vi "Digital_Bridge_3_kart.vi"() -> ()   [LabVIEW 2014] (continued)
                      frame False {
                        n3107 = local read "X Range KV"() -> (w6899:dbl)
                        n3108 = local read "Y Range KV"() -> (w6898:dbl)
                        n3109 = global write "show_sensitivity.vi" "show sensitivity (kelvin  x)"(w6899) -> ()
                        n3110 = global write "show_sensitivity.vi" "show sensitivity (kelvin  y)"(w6898) -> ()
                      }
                      frame True {
                        w6900 = 10.0 ("Max. Hassasiyet")
                        n3111 = global write "show_sensitivity.vi" "show sensitivity (kelvin  x)"(w6900) -> ()
                        n3112 = global write "show_sensitivity.vi" "show sensitivity (kelvin  y)"(w6900) -> ()
                      }
                    }
                  }
                  frame #6 {
                    n3113 = local write "kelvin switch"(FALSE ("wagner switch")) -> ()
                    n3114 = local write "Start Kelvin X"(TRUE ("START WAGNER")) -> ()
                  }
                }
              }
            }
            n3115 = case shown="True" "RESET SENS X 5" {
              frame False {
              }
              frame True {
                n3116 = local read "count meas"() -> (w6956:u16)
                n3117 = local read "iterasyon KELVIN"() -> (w6954:dbl)
                n3118 = Greater?(x=w6956, y=u16 8) -> (0:w6952:bool)
                n3119 = Greater?(x=w6954, y=5.0) -> (0:w6951:bool)
                n3120 = Or(x=w6952, y=w6951) -> (x .or. y?=w6950:bool)
                n3121 = case shown="True" w6950 {
                  frame False {
                    n3122 = flat-sequence {
                      frame #0 {
                        n3123 = global read "show_sensitivity.vi" "show sensitivity (kelvin  x)"() -> (w6957:dbl)
                        n3124 = local read "GPIB In"() -> (w6958:refnum<visa-resource-name>)
                        n3125 = call "get_sensitivity.vi"("input 1"=w6957, "SR850 GPIB In"=w6958) -> ()  [unwired: 8 in, 2 out]
                      }
                      frame #1 {
                        n3126 = Wait (ms)(milliseconds to wait=u32 500) -> ()  [unwired: 1 out]
                      }
                      frame #2 {
                        n3127 = local write "RESET SENS X 5"(FALSE ("RESET SENS X")) -> ()
                        n3128 = local write "START X 5"(TRUE ("START X 4")) -> ()
                      }
                    }
                  }
                  frame True {
                    n3129 = local read "iterasyon KELVIN"() -> (w6963:dbl)
                    n3130 = Greater?(x=w6963, y=5.0) -> (0:w6962:bool)
                    n3131 = case shown="False" w6962 {
                      frame False {
                        n3132 = flat-sequence {
                          frame #0 {
                            n3133 = local write "RESET SENS X 5"(FALSE ("Start 10R X")) -> ()
                            n3134 = local write "count meas"(u16 9 ("count meas")) -> ()
                            n3135 = local write "İterasyon X 5"(0.0 ("İterasyon X 5")) -> ()
                          }
                          frame #1 {
                            n3136 = local write "reset values"(TRUE ("Start 10R X")) -> ()
                            n3137 = local write "error"(TRUE ("Start 10R X")) -> ()
                          }
                        }
                      }
                      frame True {
                        n3138 = flat-sequence {
                          frame #0 {
                            n3139 = local write "RESET SENS X 5"(FALSE ("Start 10R X")) -> ()
                            n3140 = local write "count meas"(u16 10 ("count meas")) -> ()
                            n3141 = local write "İterasyon X 5"(0.0 ("İterasyon X 5")) -> ()
                          }
                          frame #1 {
                            n3142 = local write "reset values"(TRUE ("Start 10R X")) -> ()
                            n3143 = local write "error"(TRUE ("Start 10R X")) -> ()
                          }
                        }
                      }
                    }
                  }
                }
              }
            }
            n3144 = case shown="True" "START X 5" {
              frame False {
              }
              frame True {
                n3145 = flat-sequence {
                  frame #0 {
                    n3146 = local read "Kelvin X(k-1)"() -> (w6976:dbl)
                    n3147 = local read "Kelvin Xk"() -> (w6975:dbl)
                    n3148 = local write "input 1 x [kelvin]"(w6975) -> ()
                    n3149 = local write "input 2 x [kelvin]"(w6976) -> ()
                    n3150 = global write "DB_Global_4_kart-Test.vi" "amplitude 2/1"(w6975) -> ()
                  }
                  frame #1 {
                    n3151 = Wait (ms)(milliseconds to wait=u32 500) -> ()  [unwired: 1 out]
                  }
                  frame #2 {
                    n3152 = local write "START X 5"(FALSE ("START X 4")) -> ()
                    n3153 = local write "X 5"(TRUE ("START X")) -> ()
                  }
                  frame #3 {
                  }
                }
              }
            }
            n3154 = case shown="True" "Optimum Range 5" {
              frame False {
              }
              frame True {
                n3155 = flat-sequence {
                  frame #0 {
                    n3156 = global read "show_sensitivity.vi" "show sensitivity (kelvin  x)"() -> (w6503:dbl)
                    n3157 = local read "GPIB In"() -> (w6504:refnum<visa-resource-name>)
                    n3158 = call "get_sensitivity.vi"("input 1"=w6503, "SR850 GPIB In"=w6504) -> ()  [unwired: 8 in, 2 out]
                  }
                  frame #1 {
                    n3159 = call "set optimum range.vi"("denge degeri"=5.0) -> ("ok"=w6505:bool)  [unwired: 14 in]
                    n3160 = case shown="True" w6505 {
                      frame False {
                      }
                      frame True {
                        n3161 = local write "Optimum Range 5"(FALSE ("Optimum Range 1")) -> ()
                        n3162 = local write "PASS KELVIN"(TRUE ("PASS KELVIN")) -> ()
                      }
                    }
                  }
                }
              }
            }
            n3163 = case shown="True" "Contiune Kelvin" {
              frame False {
              }
              frame True {
                n3164 = local read "iterasyon KELVIN"() -> (w6565:dbl)
                n3165 = local read "1 or 10"() -> (w6561:i32)
                n3166 = local read "frekans index"() -> (w6560:dbl)
                n3167 = local read "control hz array"() -> (w6556:dbl[][])
                n3168 = call "change2d.vi"("reset(default false)"=FALSE, "index (col)"=w6560, "index (row)"=2, "read/write(T/F)"=TRUE, "2D Array"=w6556) -> ("result count"=w6555:dbl)  [unwired: 5 in, 1 out]
                n3169 = local read "set"() -> (w6554:u16)
                n3170 = case shown="1" w6561 {
                  tunnel: [FALSE TRUE] -> w6562
                  frame 10, Default {
                  }
                  frame 1 {
                  }
                }
                n3171 = Equal?(x=w6555, y=w6554) -> (x = y?=w6553:bool)
                n3172 = Greater?(x=w6565, y=0.0) -> (0:w6563:bool)
                n3173 = Or(x=w6563, y=w6562) -> (x .or. y?=w6552:bool)
                n3174 = Or(x=w6552, y=w6553) -> (x .or. y?=w6551:bool)
                n3175 = case shown="True" w6551 {
                  frame False {
                    n3176 = local write "Contiune Kelvin"(FALSE ("START WAGNER")) -> ()
                    n3177 = local write "RESET SENS X 5"(TRUE ("START X")) -> ()
                    n3178 = local write "Boolean 5"(FALSE ("Boolean 4")) -> ()
                  }
                  frame True {
                    n3179 = local write "Optimum Range 5"(TRUE ("START X")) -> ()
                    n3180 = local write "Contiune Kelvin"(FALSE ("Boolean 4")) -> ()
                    n3181 = local write "Boolean 5"(FALSE ("Boolean 4")) -> ()
                  }
                }
              }
            }
            n3182 = case shown="True" "PASS KELVIN" {
              frame False {
              }
              frame True {
                n3183 = flat-sequence {
                  frame #0 {
                    n3184 = Wait (ms)(milliseconds to wait=u32 3000) -> ()  [unwired: 1 out]
                  }
                  frame #1 {
                    n3185 = local read "Other Array"() -> (w6774:dbl[])
                    n3186 = for {
                      N: 7 -> [_]
                      shift-right: [w6808] -> w6777
                      shift-left: w6774 -> [w6811]
                      i -> [w6810]
                      n3187 = case shown="6" w6810 {
                        tunnel: [5.0 ("iterasyon WAGNER") w6813 w6814 w6815 w6816 w6817 w6818] -> w6809
                        frame 0, Default {
                        }
                        frame 1 {
                          n3188 = local read "Iterasyon Successful"() -> (w6813:dbl)
                        }
                        frame 2 {
                          n3189 = local read "Direnc 1 - Direnc 2"() -> (w6814:u32)
                        }
                        frame 3 {
                          n3190 = local read "olcum"() -> (w6815:u16)
                        }
                        frame 4 {
                          n3191 = local read "set"() -> (w6816:u16)
                        }
                        frame 5 {
                          n3192 = local read "frekans index"() -> (w6817:dbl)
                        }
                        frame 6 {
                          n3193 = local read "iterasyon KELVIN"() -> (w6818:dbl)
                        }
                      }
                      n3194 = Replace Array Subset(array=w6811, new element=w6809, index=w6810) -> (w6808:dbl[])
                    }
                    n3195 = local read "Output Denge Kosulu x2_y2"() -> (w6779:dbl[][])
                    n3196 = control-ref of="Default Values Listbox"() -> (w6757:refnum<vi>)
                    n3197 = local read "Output Denge Kosulu x1_x2"() -> (w6753:dbl[][])
                    n3198 = local read "Outpu Denge Kosulu y1_y2"() -> (w6752:dbl[][])
                    n3199 = local read "Frekanslar"() -> (w6739:dbl[])
                    n3200 = local read "Cluster"() -> (w6755:T2)
                    n3201 = local read "Cluster 2"() -> (w6754:T1)
                    n3202 = Array Size(array=w6739) -> (size(s)=w6738:i32)
                    n3203 = local read "input values"() -> (w6756:dbl[])
                    n3204 = call "merge_x_y.vi"("frekans size"=w6738, "y1_y2"=w6752, "x1_x2"=w6753) -> ("x1_x2_y1_y2"=w6751:dbl[][])  [unwired: 8 in]
                    n3205 = local read "default values"() -> (w6778:T3)
                    n3206 = local read "Sheet name"() -> (w6775:string)
                    n3207 = local read "Other Boolean Array"() -> (w6773:bool[])
                    n3208 = for {
                      N: 5 -> [_]
                      shift-right: [w6799] -> w6776
                      shift-left: w6773 -> [w6802]
                      i -> [w6801]
                      n3209 = case shown="1" w6801 {
                        tunnel: [FALSE FALSE FALSE FALSE FALSE] -> w6800
                        frame 0, Default {
                        }
                        frame 1 {
                        }
                        frame 2 {
                        }
                        frame 3 {
                        }
                        frame 4 {
                        }
                      }
                      n3210 = Replace Array Subset(array=w6802, new element=w6800, index=w6801) -> (w6799:bool[])
                    }
                    n3211 = call "Pass.vi"("Other Array"=w6777, "Other Boolean Array"=w6776, "Denge Kosulu x2_y2"=w6779, "LstBox Refnum"=w6757, "Cluster"=w6755, "F/P Array Cluster"=w6754, "Sheet name"=w6775, "default values"=w6778, "x1_x2_y1_y2"=w6751, "input values"=w6756) -> ("output values"=w6750:dbl[], "Output Other Boolean Array"=w6770:bool[], "Output Cluster"=w6749:T2, "Output F/P Array Cluster"=w6745:T1, "output default values"=w6772:T11, "Output Iterasyon Successful"=w6771:dbl, "Denge Seçimi"=w6759:u8, "end time"=w6758:string)  [unwired: 1 in, 1 out]
                    n3212 = local write "input values"(w6750) -> ()
                    n3213 = Unbundle By Name(w6749) -> ("F Values Array"=w6748:dbl[][], "control hz array"=w6747:dbl[][], "extra default values"=w6746:dbl[][])
                    n3214 = Unbundle By Name(w6745) -> ("AD F/P Array"=w6740:dbl[][], "10R F/P Array"=w6741:dbl[][], "1R F/P Array"=w6742:dbl[][], "Wagner F/P Array"=w6743:dbl[][], "Kelvin F/P Array"=w6744:dbl[][])
                    n3215 = local write "default values"(w6772) -> ()
                    n3216 = local write "Iterasyon Successful"(w6771) -> ()
                    n3217 = local write "AD F/P Array"(w6740) -> ()
                    n3218 = local write "10R F/P Array"(w6741) -> ()
                    n3219 = local write "1R F/P Array"(w6742) -> ()
                    n3220 = local write "Wagner F/P Array"(w6743) -> ()
                    n3221 = local write "Kelvin F/P Array"(w6744) -> ()
                    n3222 = local write "F Values Array"(w6748) -> ()
                    n3223 = local write "control hz array"(w6747) -> ()
                    n3224 = local write "extra default values"(w6746) -> ()
                    n3225 = Index Array(array=w6770, index #1=0 ("index"), index #2=1 ("index"), index #3=2 ("index"), index #4=3 ("index"), index #5=4 ("index")) -> (element #1=w6764:bool, element #2=w6763:bool, element #3=w6762:bool, element #4=w6761:bool, element #5=w6760:bool)
                    n3226 = case shown="True" w6764 {
                      frame False {
                      }
                      frame True {
                        n3227 = local write "PASS KELVIN"(FALSE ("PASS KELVIN")) -> ()
                        n3228 = local write "reset values"(TRUE ("reset values")) -> ()
                        n3229 = local write "Boolean 5"(TRUE ("Boolean 4")) -> ()
                        n3230 = local write "pass hz"(TRUE ("pass hz")) -> ()
                      }
                    }
                    n3231 = case shown="True" w6763 {
                      tunnel: w6759 -> [_ w6793]
                      frame False {
                      }
                      frame True {
                        n3232 = local write "Ana denge Switch"(TRUE ("10R switch")) -> ()
                        n3233 = local write "PASS KELVIN"(FALSE ("PASS KELVIN")) -> ()
                        n3234 = local write "Denge Seçimi"(w6793) -> ()
                        n3235 = local write "count meas"(u16 0 ("count meas")) -> ()
                        n3236 = local write "Boolean 5"(TRUE ("Boolean 4")) -> ()
                      }
                    }
                    n3237 = case shown="True" w6762 {
                      tunnel: w6758 -> [_ w6788]
                      frame False {
                      }
                      frame True {
                        n3238 = local write "PASS KELVIN"(FALSE ("PASS KELVIN")) -> ()
                        n3239 = local write "reset values"(TRUE ("reset values")) -> ()
                        n3240 = local write "end time"(w6788) -> ()
                        n3241 = local write "Boolean 5"(TRUE ("Boolean 4")) -> ()
                      }
                    }
                    n3242 = case shown="True" w6761 {
                      frame False {
                      }
                      frame True {
                        n3243 = local write "RESET SENS X 5"(TRUE ("RESET SENS X 4")) -> ()
                        n3244 = local write "PASS KELVIN"(FALSE ("PASS KELVIN")) -> ()
                      }
                    }
                    n3245 = case shown="True" w6760 {
                      frame False {
                      }
                      frame True {
                        n3246 = local write "RESET SENS Y 5"(TRUE ("RESET SENS Y 4")) -> ()
                        n3247 = local write "PASS KELVIN"(FALSE ("PASS KELVIN")) -> ()
                      }
                    }
                  }
                  frame #2 {
                  }
                }
              }
            }
            n3248 = case shown="True" "auto phase kelvin" {
              frame False {
              }
              frame True {
                n3249 = flat-sequence {
                  frame #0 {
                    n3250 = local read "GPIB In"() -> (w6822:refnum<visa-resource-name>)
                    n3251 = local read "GPIB In"() -> (w6820:refnum<visa-resource-name>)
                    n3252 = call "Reserve.vi"("Reserve(MAX-MIN)"="2", "VISA resource name"=w6820) -> ()  [unwired: 8 in, 2 out]
                    n3253 = call "reference phase.vi"("Reference Phase (0.000 degrees)"="0", "VISA resource name"=w6822) -> ()  [unwired: 8 in, 2 out]
                  }
                  frame #1 {
                    w6824 = u16 0 items=["100 nV", "200 nV", "500 nV", "1 uV", "2 uV", "5 uV", "10 uV", "20 uV", "50 uV", "100 uV", "200 uV", "500 uV", "1 mV"] ("Min. Hassasiyet")
                    n3254 = local read "X Range KV"() -> (w6823:dbl)
                    n3255 = local read "GPIB In"() -> (w6825:refnum<visa-resource-name>)
                    n3256 = call "GAIN BASIC.vi"("SR850 GPIB In"=w6825, "Max. Hassasiyet"=w6823, "Auto Gain (False)"=FALSE, "Min. Hassasiyet"=w6824) -> ()  [unwired: 10 in, 2 out]
                  }
                  frame #2 {
                    n3257 = local read "X 1.input KV"() -> (w6827:dbl)
                    n3258 = global write "DB_Global_4_kart-Test.vi" "amplitude 2/1"(w6827) -> ()
                    n3259 = global write "DB_Global_4_kart-Test.vi" "phase 2/1"(w6827) -> ()
                  }
                  frame #3 {
                    n3260 = Wait (ms)(milliseconds to wait=u32 750) -> ()  [unwired: 1 out]
                  }
                  frame #4 {
                    n3261 = local write "read x1 y1 5"(TRUE ("output x")) -> ()
                    n3262 = local write "auto phase kelvin"(FALSE ("auto phase wagner")) -> ()
                  }
                }
              }
            }
            n3263 = case shown="True" "RANGE KONTROL Y 5" {
              frame False {
              }
              frame True {
                n3264 = local read "Outpu Denge Kosulu y1_y2"() -> (w6613:dbl[][])
                n3265 = local read "iterasyon KELVIN"() -> (w6612:dbl)
                n3266 = local read "input 1 y [kelvin]"() -> (w6614:dbl)
                n3267 = local read "frekans index"() -> (w6606:dbl)
                n3268 = local read "input 2 y [kelvin]"() -> (w6615:dbl)
                n3269 = local read "output 2 y [kelvin]"() -> (w6609:dbl)
                n3270 = local read "output 1 y [kelvin]"() -> (w6611:dbl)
                n3271 = call "Range Kontrol Y.vi"("denge degeri"=5.0, "iterasyon Denge"=w6612, "frekans index"=w6606, "Denge Kosulu y1_y2"=w6613, "Yk"=w6614, "Y(k-1)"=w6615, "output y 1"=w6611, "output y 2"=w6609) -> ("Output Y(k-1)"=w6605:dbl, "result output y"=w6616:dbl, "KONTROL X"=w6608:bool, "IF ELSE"=w6607:bool)  [unwired: 8 in]
                n3272 = local write "Kelvin Y(k-1)"(w6605) -> ()
                n3273 = local write "result output y [Kelvin]"(w6616) -> ()
                n3274 = flat-sequence {
                  tunnel: w6608 -> [w6618]
                  tunnel: w6607 -> [w6617]
                  frame #0 {
                    n3275 = case shown="True" w6617 {
                      frame False {
                      }
                      frame True {
                        n3276 = local write "IF ELSE Y 5"(TRUE ("IF ELSE X 4")) -> ()
                      }
                    }
                    n3277 = case shown="True" w6618 {
                      frame False {
                      }
                      frame True {
                        n3278 = local write "KONTROL X 5"(TRUE ("KONTROL Y 4")) -> ()
                      }
                    }
                  }
                  frame #1 {
                    n3279 = local write "RANGE KONTROL Y 5"(FALSE ("KONTROL Y 4")) -> ()
                    n3280 = local read "İterasyon Y 5"() -> (w6621:dbl)
                    n3281 = Increment(x=w6621) -> (x+1=w6622:dbl)
                    n3282 = local write "İterasyon Y 5"(w6622) -> ()
                  }
                }
              }
            }
            n3283 = case shown="True" "RANGE KONTROL X 5" {
              frame False {
              }
              frame True {
                n3284 = local read "Output Denge Kosulu x1_x2"() -> (w6694:dbl[][])
                n3285 = local read "iterasyon KELVIN"() -> (w6693:dbl)
                n3286 = local read "input 1 x [kelvin]"() -> (w6695:dbl)
                n3287 = local read "frekans index"() -> (w6686:dbl)
                n3288 = local read "input 2 x [kelvin]"() -> (w6696:dbl)
                n3289 = local read "output 2 x [kelvin]"() -> (w6690:dbl)
                n3290 = local read "output 1 x [kelvin]"() -> (w6692:dbl)
                n3291 = call "Range Kontrol X.vi"("denge degeri"=5.0, "iterasyon Denge"=w6693, "frekans index"=w6686, "Denge Kosulu x1_x2"=w6694, "Xk"=w6695, "X(k-1)"=w6696, "output x 1"=w6692, "output x 2"=w6690) -> ("Output X(k-1)"=w6685:dbl, "result output x"=w6697:dbl, "KONTROL Y"=w6689:bool, "IF ELSE"=w6688:bool, "Start Denge Y"=w6687:bool)  [unwired: 7 in]
                n3292 = local write "Kelvin X(k-1)"(w6685) -> ()
                n3293 = local write "result output x [Kelvin]"(w6697) -> ()
                n3294 = flat-sequence {
                  tunnel: w6689 -> [w6700]
                  tunnel: w6688 -> [w6699]
                  tunnel: w6687 -> [w6698]
                  frame #0 {
                    n3295 = case shown="True" w6698 {
                      frame False {
                      }
                      frame True {
                        n3296 = local write "Start Kelvin Y"(TRUE ("Start Wagner Y")) -> ()
                      }
                    }
                    n3297 = case shown="True" w6699 {
                      frame False {
                      }
                      frame True {
                        n3298 = local write "IF ELSE X 5"(TRUE ("IF ELSE X 4")) -> ()
                      }
                    }
                    n3299 = case shown="True" w6700 {
                      frame False {
                      }
                      frame True {
                        n3300 = local write "KONTROL Y 5"(TRUE ("KONTROL Y 4")) -> ()
                      }
                    }
                  }
                  frame #1 {
                    n3301 = local write "RANGE KONTROL X 5"(FALSE ("KONTROL Y 4")) -> ()
                    n3302 = local read "İterasyon X 5"() -> (w6705:dbl)
                    n3303 = Increment(x=w6705) -> (x+1=w6704:dbl)
                    n3304 = local write "İterasyon X 5"(w6704) -> ()
                  }
                }
              }
            }
            n3305 = case shown="True" "Y 5" {
              frame False {
              }
              frame True {
                n3306 = local read "İterasyon Y 5"() -> (w6645:dbl)
                n3307 = local read "Kelvin Y(k-1)"() -> (w6646:dbl)
                n3308 = call "Y.vi"("Y(k-1)"=w6646, "İterasyon Denge"=w6645, "denge degeri"=5.0) -> ("error"=w6643:bool, "output Y(k-1)"=w6640:dbl, "output y 1"=w6641:dbl, "cycle"=w6642:bool)  [unwired: 5 in]
                n3309 = case shown="False" w6642 {
                  tunnel: w6643 -> [w6649 _]
                  tunnel: w6641 -> [w6648 _]
                  tunnel: w6640 -> [w6647 _]
                  frame False {
                    n3310 = case shown="False" w6649 {
                      frame False {
                        n3311 = local write "Y1 5"(TRUE ("X1 4")) -> ()
                        n3312 = local write "Y 5"(FALSE ("X 4")) -> ()
                      }
                      frame True {
                        n3313 = local write "error"(TRUE ("X1 4")) -> ()
                        n3314 = local write "Y 5"(FALSE ("X 4")) -> ()
                      }
                    }
                    n3315 = local write "output 1 y [kelvin]"(w6648) -> ()
                    n3316 = local write "Kelvin Y(k-1)"(w6647) -> ()
                    n3317 = local write "input 2 y [kelvin]"(w6647) -> ()
                  }
                  frame True {
                  }
                }
              }
            }
            n3318 = case shown="True" "X 5" {
              frame False {
              }
              frame True {
                n3319 = local read "İterasyon X 5"() -> (w6728:dbl)
                n3320 = local read "Kelvin X(k-1)"() -> (w6729:dbl)
                n3321 = call "X.vi"("X(k-1)"=w6729, "İterasyon Denge"=w6728, "denge degeri"=5.0) -> ("error"=w6726:bool, "output X(k-1)"=w6723:dbl, "output x 1"=w6724:dbl, "cycle"=w6725:bool)  [unwired: 5 in]
                n3322 = case shown="False" w6725 {
                  tunnel: w6726 -> [w6732 _]
                  tunnel: w6724 -> [w6731 _]
                  tunnel: w6723 -> [w6730 _]
                  frame False {
                    n3323 = case shown="False" w6732 {
                      frame False {
                        n3324 = local write "X1 5"(TRUE ("X1 4")) -> ()
                        n3325 = local write "X 5"(FALSE ("X 4")) -> ()
                      }
                      frame True {
                        n3326 = local write "error"(TRUE ("X1 4")) -> ()
                        n3327 = local write "X 5"(FALSE ("X 4")) -> ()
                      }
                    }
                    n3328 = local write "output 1 x [kelvin]"(w6731) -> ()
                    n3329 = local write "Kelvin X(k-1)"(w6730) -> ()
                    n3330 = local write "input 2 x [kelvin]"(w6730) -> ()
                  }
                  frame True {
                  }
                }
              }
            }
            n3331 = case shown="True" "read x1 y1 5" {
              frame False {
              }
              frame True {
                n3332 = local read "X Range KV"() -> (w6487:dbl)
                n3333 = call "only_x_and_y_output.vi"("range"=w6487) -> ("cycle 2"=w6491:bool, "range 2"=w6488:dbl, "Output Y"=w6489:dbl, "Output X"=w6490:dbl)  [unwired: 7 in]
                n3334 = case shown="False" w6491 {
                  tunnel: w6490 -> [w6494 _]
                  tunnel: w6489 -> [w6493 _]
                  tunnel: w6488 -> [w6492 w6502]
                  frame False {
                    n3335 = flat-sequence {
                      tunnel: w6494 -> [w6497]
                      tunnel: w6493 -> [w6496]
                      tunnel: w6492 -> [w6495]
                      frame #0 {
                        n3336 = local write "X Range KV"(w6495) -> ()
                        n3337 = local write "Output Y1"(w6496) -> ()
                        n3338 = local write "Output X1"(w6497) -> ()
                      }
                      frame #1 {
                        n3339 = local read "X 2.input KV"() -> (w6498:dbl)
                        n3340 = global write "DB_Global_4_kart-Test.vi" "amplitude 2/1"(w6498) -> ()
                      }
                      frame #2 {
                        n3341 = Wait (ms)(milliseconds to wait=u32 750) -> ()  [unwired: 1 out]
                      }
                      frame #3 {
                        n3342 = local write "read x1 y1 5"(FALSE ("output x")) -> ()
                        n3343 = local write "read x2 y2 5"(TRUE ("output x")) -> ()
                      }
                    }
                  }
                  frame True {
                    n3344 = local write "X Range KV"(w6502) -> ()
                  }
                }
              }
            }
            n3345 = case shown="True" "Y1 5" {
              frame False {
              }
              frame True {
                n3346 = local read "output 1 y [kelvin]"() -> (w6632:dbl)
                n3347 = local read "İterasyon Y 5"() -> (w6629:dbl)
                n3348 = local read "Kelvin Y(k-1)"() -> (w6631:dbl)
                n3349 = local read "Kelvin Yk"() -> (w6630:dbl)
                n3350 = call "Y1.vi"("denge degeri"=5.0, "İterasyon Denge"=w6629, "Yk"=w6630, "Y(k-1)"=w6631, "output y 1"=w6632) -> ("Output Yk"=w6625:dbl, "output y 2"=w6624:dbl, "cycle"=w6626:bool, "error"=w6627:bool)  [unwired: 7 in]
                n3351 = case shown="False" w6626 {
                  tunnel: w6627 -> [w6635 _]
                  tunnel: w6625 -> [w6634 _]
                  tunnel: w6624 -> [w6633 _]
                  frame False {
                    n3352 = case shown="True" w6635 {
                      frame False {
                        n3353 = local write "RANGE KONTROL Y 5"(TRUE ("RANGE KONTROL X 4")) -> ()
                        n3354 = local write "Y1 5"(FALSE ("X1 4")) -> ()
                      }
                      frame True {
                        n3355 = local write "error"(TRUE ("RANGE KONTROL X 4")) -> ()
                        n3356 = local write "Y1 5"(FALSE ("X1 4")) -> ()
                      }
                    }
                    n3357 = local write "Kelvin Yk"(w6634) -> ()
                    n3358 = local write "output 2 y [kelvin]"(w6633) -> ()
                  }
                  frame True {
                  }
                }
              }
            }
            n3359 = case shown="True" "X1 5" {
              frame False {
              }
              frame True {
                n3360 = local read "output 1 x [kelvin]"() -> (w6715:dbl)
                n3361 = local read "İterasyon X 5"() -> (w6712:dbl)
                n3362 = local read "Kelvin X(k-1)"() -> (w6714:dbl)
                n3363 = local read "Kelvin Xk"() -> (w6713:dbl)
                n3364 = call "X1.vi"("denge degeri"=5.0, "İterasyon Denge"=w6712, "Xk"=w6713, "X(k-1)"=w6714, "output x 1"=w6715) -> ("Output Xk"=w6707:dbl, "output x 2"=w6708:dbl, "cycle"=w6709:bool, "error"=w6710:bool)  [unwired: 7 in]
                n3365 = case shown="False" w6709 {
                  tunnel: w6710 -> [w6718 _]
                  tunnel: w6708 -> [w6717 _]
                  tunnel: w6707 -> [w6716 _]
                  frame False {
                    n3366 = case shown="False" w6718 {
                      frame False {
                        n3367 = local write "RANGE KONTROL X 5"(TRUE ("RANGE KONTROL X 4")) -> ()
                        n3368 = local write "X1 5"(FALSE ("X1 4")) -> ()
                      }
                      frame True {
                        n3369 = local write "error"(TRUE ("RANGE KONTROL X 4")) -> ()
                        n3370 = local write "X1 5"(FALSE ("X1 4")) -> ()
                      }
                    }
                    n3371 = local write "Kelvin Xk"(w6716) -> ()
                    n3372 = local write "output 2 x [kelvin]"(w6717) -> ()
                  }
                  frame True {
                  }
                }
              }
            }
            n3373 = case shown="True" "IF ELSE Y 5" {
              frame False {
              }
              frame True {
                n3374 = local read "input 1 y [kelvin]"() -> (w6594:dbl)
                n3375 = local read "input 2 y [kelvin]"() -> (w6595:dbl)
                n3376 = local read "output 1 y [kelvin]"() -> (w6598:dbl)
                n3377 = local read "result output y [Kelvin]"() -> (w6600:dbl)
                n3378 = local read "output 2 y [kelvin]"() -> (w6599:dbl)
                n3379 = call "If Else Y.vi"("denge degeri"=5.0, "Yk"=w6594, "Y(k-1)"=w6595, "output y 1"=w6598, "output y 2"=w6599, "result output y"=w6600) -> ("Output Y(k-1)"=w6593:dbl, "Start Y"=w6596:bool)  [unwired: 8 in]
                n3380 = local write "Kelvin Y(k-1)"(w6593) -> ()
                n3381 = case shown="True" w6596 {
                  frame False {
                  }
                  frame True {
                    n3382 = local read "count meas"() -> (w6602:u16)
                    n3383 = local write "RESET SENS Y 5"(TRUE ("START X 4")) -> ()
                    n3384 = Increment(x=w6602) -> (x+1=w6601:u16)
                    n3385 = local write "count meas"(w6601) -> ()
                    n3386 = local write "IF ELSE Y 5"(FALSE ("IF ELSE X 4")) -> ()
                  }
                }
              }
            }
            n3387 = case shown="True" "IF ELSE X 5" {
              frame False {
              }
              frame True {
                n3388 = local read "input 1 x [kelvin]"() -> (w6674:dbl)
                n3389 = local read "input 2 x [kelvin]"() -> (w6675:dbl)
                n3390 = local read "output 1 x [kelvin]"() -> (w6678:dbl)
                n3391 = local read "result output x [Kelvin]"() -> (w6680:dbl)
                n3392 = local read "output 2 x [kelvin]"() -> (w6679:dbl)
                n3393 = call "If Else X.vi"("denge degeri"=5.0, "Xk"=w6674, "X(k-1)"=w6675, "output x 1"=w6678, "output x 2"=w6679, "result output x"=w6680) -> ("Output X(k-1)"=w6673:dbl, "Start X"=w6676:bool)  [unwired: 8 in]
                n3394 = local write "Kelvin X(k-1)"(w6673) -> ()
                n3395 = case shown="True" w6676 {
                  frame False {
                  }
                  frame True {
                    n3396 = local read "count meas"() -> (w6681:u16)
                    n3397 = local write "RESET SENS X 5"(TRUE ("START X 4")) -> ()
                    n3398 = local write "IF ELSE X 5"(FALSE ("IF ELSE X 4")) -> ()
                    n3399 = Increment(x=w6681) -> (x+1=w6682:u16)
                    n3400 = local write "count meas"(w6682) -> ()
                  }
                }
              }
            }
            n3401 = case shown="True" "read x2 y2 5" {
              frame False {
              }
              frame True {
                n3402 = local read "X Range KV"() -> (w6471:dbl)
                n3403 = call "only_x_and_y_output.vi"("range"=w6471) -> ("cycle 2"=w6475:bool, "range 2"=w6472:dbl, "Output Y"=w6473:dbl, "Output X"=w6474:dbl)  [unwired: 7 in]
                n3404 = case shown="False" w6475 {
                  tunnel: w6474 -> [w6478 _]
                  tunnel: w6473 -> [w6477 _]
                  tunnel: w6472 -> [w6476 w6486]
                  frame False {
                    n3405 = flat-sequence {
                      tunnel: w6478 -> [w6481]
                      tunnel: w6477 -> [w6480]
                      tunnel: w6476 -> [w6479]
                      frame #0 {
                        n3406 = local write "Output X2"(w6481) -> ()
                        n3407 = local write "Output Y2"(w6480) -> ()
                        n3408 = local write "X Range KV"(w6479) -> ()
                      }
                      frame #1 {
                        n3409 = global write "DB_Global_4_kart-Test.vi" "amplitude 2/1"(0.0) -> ()
                      }
                      frame #2 {
                        n3410 = Wait (ms)(milliseconds to wait=u32 750) -> ()  [unwired: 1 out]
                      }
                      frame #3 {
                        n3411 = local write "result phase 5"(TRUE ("result phase 4")) -> ()
                        n3412 = local write "read x2 y2 5"(FALSE ("output y")) -> ()
                      }
                    }
                  }
                  frame True {
                    n3413 = local write "X Range KV"(w6486) -> ()
                  }
                }
              }
            }
            n3414 = case shown="True" "KONTROL X 5" {
              frame False {
              }
              frame True {
                n3415 = local read "Output Denge Kosulu x1_x2"() -> (w6582:dbl[][])
                n3416 = local read "iterasyon KELVIN"() -> (w6574:dbl)
                n3417 = local read "Manuel/Otomatik"() -> (w6581:enum16{"Manuel", "Otomatik"})
                n3418 = local read "frekans index"() -> (w6575:dbl)
                n3419 = call "Kontrol X.vi"("denge degeri"=5.0, "İterasyon Denge"=w6574, "Denge Kosulu x1_x2"=w6582, "Manuel/Otomatik"=w6581, "frekans index"=w6575) -> ("Denge Seçimi"=w6578:u8, "New İterasyon Denge"=w6577:dbl, "Iterasyon Count Successful"=w6576:dbl, "Start Denge X"=w6579:bool)  [unwired: 7 in]
                n3420 = case shown="True" w6579 {
                  tunnel: w6578 -> [w6590 _]
                  tunnel: w6577 -> [_ _]
                  tunnel: w6576 -> [w6589 _]
                  frame False {
                    n3421 = local write "Iterasyon Successful"(w6589) -> ()
                    n3422 = local write "Ana denge Switch"(TRUE ("10R switch")) -> ()
                    n3423 = local write "count meas"(u16 0 ("count meas")) -> ()
                    n3424 = local write "Denge Seçimi"(w6590) -> ()
                    n3425 = local read "iterasyon KELVIN"() -> (w6584:dbl)
                    n3426 = local write "Boolean 5"(TRUE ("Boolean 4")) -> ()
                    n3427 = local write "KONTROL X 5"(FALSE ("KONTROL X 5")) -> ()
                    n3428 = Increment(x=w6584) -> (x+1=w6583:dbl)
                    n3429 = local write "iterasyon KELVIN"(w6583) -> ()
                  }
                  frame True {
                    n3430 = local write "KONTROL X 5"(FALSE ("KONTROL X 5")) -> ()
                    n3431 = local write "RESET SENS X 5"(TRUE ("Start Wagner Y")) -> ()
                  }
                }
              }
            }
            n3432 = case shown="True" "KONTROL Y 5" {
              frame False {
              }
              frame True {
                n3433 = local read "Outpu Denge Kosulu y1_y2"() -> (w6662:dbl[][])
                n3434 = local read "iterasyon KELVIN"() -> (w6654:dbl)
                n3435 = local read "Manuel/Otomatik"() -> (w6661:enum16{"Manuel", "Otomatik"})
                n3436 = local read "frekans index"() -> (w6655:dbl)
                n3437 = call "Kontrol Y.vi"("denge degeri"=5.0, "İterasyon Denge"=w6654, "Denge Kosulu y1_y2"=w6662, "Manuel/Otomatik"=w6661, "frekans index"=w6655) -> ("Denge Seçimi"=w6658:u8, "New İterasyon Denge"=w6657:dbl, "Iterasyon Count Successful"=w6656:dbl, "Start Denge Y"=w6659:bool)  [unwired: 7 in]
                n3438 = case shown="True" w6659 {
                  tunnel: w6658 -> [w6670 _]
                  tunnel: w6657 -> [_ _]
                  tunnel: w6656 -> [w6669 _]
                  frame False {
                    n3439 = local write "count meas"(u16 0 ("count meas")) -> ()
                    n3440 = local write "Iterasyon Successful"(w6669) -> ()
                    n3441 = local write "Ana denge Switch"(TRUE ("10R switch")) -> ()
                    n3442 = local write "Denge Seçimi"(w6670) -> ()
                    n3443 = local read "iterasyon KELVIN"() -> (w6664:dbl)
                    n3444 = local write "KONTROL Y 5"(FALSE ("KONTROL Y 5")) -> ()
                    n3445 = local write "Boolean 5"(TRUE ("Boolean 4")) -> ()
                    n3446 = Increment(x=w6664) -> (x+1=w6663:dbl)
                    n3447 = local write "iterasyon KELVIN"(w6663) -> ()
                  }
                  frame True {
                    n3448 = local write "RESET SENS Y 5"(TRUE ("Start Wagner Y")) -> ()
                    n3449 = local write "KONTROL Y 5"(FALSE ("KONTROL Y 5")) -> ()
                  }
                }
              }
            }
            n3450 = case shown="True" "result phase 5" {
              frame False {
              }
              frame True {
                n3451 = flat-sequence {
                  tunnel: [w6516] -> w6511
                  tunnel: w6511 -> [w6532]
                  tunnel: [w6532] -> w6510
                  tunnel: w6510 -> [w6537]
                  tunnel: [w6537] -> w6509
                  tunnel: w6509 -> [w6543]
                  frame #0 {
                    # "pi"
                    n3452 = local read "Output X1"() -> (w6515:dbl)
                    n3453 = local read "Output X2"() -> (w6514:dbl)
                    n3454 = local read "Output Y1"() -> (w6513:dbl)
                    n3455 = local read "Output Y2"() -> (w6512:dbl)
                    n3456 = local read "GPIB In"() -> (w6521:refnum<visa-resource-name>)
                    n3457 = call "return phase.vi"("VISA resource name"=w6521) -> ("return phase"=w6517:string)  [unwired: 10 in]
                    n3458 = Fract/Exp String To Number(use system decimal point (T)=FALSE, string=w6517) -> (number=w6519:dbl)  [unwired: 2 in, 1 out]
                    n3459 = formula code="theta = atan((y2-y1)/(x2-x1))*(180/pi)+phase;"("x1"=w6515, "x2"=w6514, "y1"=w6513, "y2"=w6512, "phase"=w6519, "pi"=3.141592653589793) -> ("theta"=w6516:dbl)
                  }
                  frame #1 {
                    n3460 = local read "frekans index"() -> (w6528:dbl)
                    n3461 = local read "Frekanslar"() -> (w6527:dbl[])
                    n3462 = local read "Cluster 2"() -> (w6524:T1)
                    n3463 = local read "Direnc 1 - Direnc 2"() -> (w6534:u32)
                    n3464 = property on="Default Values Listbox" class="LstBox (strict)"() -> ("Item Names"=w6526:string[])  [unwired: 2 in, 2 out]
                    n3465 = Fract/Exp String To Number(string=w6526) -> (number=w6529:dbl[])  [unwired: 3 in, 1 out]
                    n3466 = Index Array(array=w6527, index=w6528) -> (element=w6531:dbl)
                    n3467 = local read "Kelvin F/P Array"() -> (w6535:dbl[][])
                    n3468 = Search 1D Array(1D array=w6529, element=w6531, start index (0)=0) -> (index of element=w6525:i32)
                    n3469 = Increment(x=w6534) -> (x+1=w6533:u32)
                    n3470 = Replace Array Subset(array=w6535, new element=w6532, index (row)=w6533, index (col)=w6525) -> (w6522:dbl[][])
                    n3471 = Bundle By Name(cluster=w6524, "Kelvin F/P Array"=w6522) -> (w6523:T1)
                    n3472 = local write "Kelvin F/P Array"(w6522) -> ()
                    n3473 = local write "Cluster 2"(w6523) -> ()
                  }
                  frame #2 {
                    n3474 = Wait (ms)(milliseconds to wait=u32 250) -> ()  [unwired: 1 out]
                  }
                  frame #3 {
                    w6540 = u16 1 items=["A", "A-B"] ("Input Source (0: A)")
                    n3475 = local read "GPIB In"() -> (w6539:refnum<visa-resource-name>)
                    n3476 = Number To Fractional String(number=w6543) -> (F-format string=w6544:string)  [unwired: 3 in]
                    n3477 = Search and Replace String(input string=w6544, search string=",", replace string="." ("replace string (\"\")")) -> (result string=w6538:string)  [unwired: 5 in, 3 out]
                    n3478 = call "reference phase.vi"("Reference Phase (0.000 degrees)"=w6538, "VISA resource name"=w6539) -> ("error out"=w6541:errorcluster, "VISA resource name out"=w6542:refnum<visa-resource-name>)  [unwired: 8 in]
                    n3479 = call "input source.vi"("error in (no error)"=w6541, "Input Source (0: A)"=w6540, "VISA resource name"=w6542) -> ()  [unwired: 7 in, 2 out]
                  }
                  frame #4 {
                    n3480 = local read "GPIB In"() -> (w6548:refnum<visa-resource-name>)
                    n3481 = local write "Contiune Kelvin"(TRUE ("Contiune Wagner")) -> ()
                    n3482 = local write "result phase 5"(FALSE ("result phase 4")) -> ()
                    n3483 = call "Reserve.vi"("Reserve(MAX-MIN)"="0", "VISA resource name"=w6548) -> ()  [unwired: 8 in, 2 out]
                  }
                }
              }
            }
          }
        }
        n3484 = local read "first process"() -> (w614:bool)
        n3485 = local read "reset values"() -> (w620:bool)
        n3486 = case shown="True" w620 {
          frame False {
          }
          frame True {
            n3487 = flat-sequence {
              frame #0 {
              }
              frame #1 {
                n3488 = local read "pass hz"() -> (w1785:bool)
                n3489 = case shown="False" w1785 {
                  frame False {
                    n3490 = local read "error 2"() -> (w1786:bool)
                    n3491 = case shown="False" w1786 {
                      frame False {
                        n3492 = local read "frekans index"() -> (w1788:dbl)
                        n3493 = local read "control hz array"() -> (w1794:dbl[][])
                        n3494 = local read "olcum"() -> (w1790:u16)
                        n3495 = call "change2d.vi"("reset(default false)"=FALSE, "index (col)"=w1788, "index (row)"=1, "read/write(T/F)"=TRUE, "2D Array"=w1794) -> ("result count"=w1791:dbl)  [unwired: 5 in, 1 out]
                        n3496 = Greater Or Equal?(x=w1791, y=w1790) -> (x >= y?=w1789:bool)
                        n3497 = case shown="True" w1789 {
                          frame False {
                            n3498 = local write "default input"(FALSE ("default values 2")) -> ()
                            n3499 = local write "continue"(TRUE ("continue")) -> ()
                          }
                          frame True {
                            n3500 = local read "Frekanslar"() -> (w1799:dbl[])
                            n3501 = Array Size(array=w1799) -> (size(s)=w1798:i32)
                            n3502 = local read "frekans index"() -> (w1800:dbl)
                            n3503 = Decrement(x=w1798) -> (x-1=w1797:i32)
                            n3504 = Equal?(x=w1800, y=w1797) -> (x = y?=w1801:bool)
                            n3505 = case shown="True" w1801 {
                              tunnel: w1800 -> [w1802 w1827]
                              frame False {
                                n3506 = flat-sequence {
                                tunnel: w1802 -> [w1805]
                                tunnel: w1802 -> [w1810]
                                frame #0 {
                                n3507 = local read "control hz array"() -> (w1807:dbl[][])
                                n3508 = call "change2d.vi"("reset(default false)"=TRUE, "index (col)"=w1805, "index (row)"=1, "read/write(T/F)"=FALSE, "2D Array"=w1807) -> ("2D Array Result"=w1808:dbl[][])  [unwired: 5 in, 1 out]
                                n3509 = local write "control hz array"(w1808) -> ()
                                }
                                frame #1 {
                                n3510 = Wait (ms)(milliseconds to wait=u32 500) -> ()  [unwired: 1 out]
                                }
                                frame #2 {
                                n3511 = local read "control hz array"() -> (w1814:dbl[][])
                                n3512 = call "change2d.vi"("reset(default false)"=FALSE, "index (col)"=w1810, "index (row)"=2, "read/write(T/F)"=FALSE, "2D Array"=w1814) -> ("2D Array Result"=w1815:dbl[][])  [unwired: 5 in, 1 out]
                                n3513 = local write "control hz array"(w1815) -> ()
                                }
                                frame #3 {
                                n3514 = local read "frekans index"() -> (w1819:dbl)
                                n3515 = local write "default input"(TRUE ("default values 2")) -> ()
                                n3516 = local write "continue"(FALSE ("continue")) -> ()
                                n3517 = Increment(x=w1819) -> (x+1=w1818:dbl)
                                n3518 = local write "frekans index"(w1818) -> ()
                                }
                                frame #4 {
                                n3519 = Multiply(x="delay f", y=u32 1000) -> (x*y=w1821:u32)
                                n3520 = Wait (ms)(milliseconds to wait=w1821) -> ()  [unwired: 1 out]
                                }
                                }
                              }
                              frame True {
                                n3521 = local read "frekans index"() -> (w1825:dbl)
                                n3522 = local read "control hz array"() -> (w1826:dbl[][])
                                n3523 = local read "set"() -> (w1824:u16)
                                n3524 = call "find 2d boolean.vi"("set"=w1824, "frekans index"=w1825, "2D Array"=w1826) -> ("logical AND"=w1823:bool)  [unwired: 8 in]
                                n3525 = case shown="True" w1823 {
                                tunnel: w1827 -> [w1829 w1851]
                                tunnel: w1827 -> [w1828 w1850]
                                frame False {
                                n3526 = flat-sequence {
                                tunnel: w1829 -> [w1830]
                                tunnel: w1828 -> [w1837]
                                frame #0 {
                                n3527 = local read "control hz array"() -> (w1833:dbl[][])
                                n3528 = call "change2d.vi"("reset(default false)"=TRUE, "index (col)"=w1830, "index (row)"=1, "read/write(T/F)"=FALSE, "2D Array"=w1833) -> ("2D Array Result"=w1834:dbl[][])  [unwired: 5 in, 1 out]
                                n3529 = local write "control hz array"(w1834) -> ()
                                }
                                frame #1 {
                                n3530 = Wait (ms)(milliseconds to wait=u32 500) -> ()  [unwired: 1 out]
                                }
                                frame #2 {
                                n3531 = local read "control hz array"() -> (w1840:dbl[][])
                                n3532 = call "change2d.vi"("reset(default false)"=FALSE, "index (col)"=w1837, "index (row)"=2, "read/write(T/F)"=FALSE, "2D Array"=w1840) -> ("2D Array Result"=w1841:dbl[][])  [unwired: 5 in, 1 out]
                                n3533 = local write "control hz array"(w1841) -> ()
                                }
                                frame #3 {
                                n3534 = local write "default input"(TRUE ("default values 2")) -> ()
                                n3535 = local write "frekans index"(0.0 ("frekans index")) -> ()
                                n3536 = local write "continue"(FALSE ("continue")) -> ()
                                }
                                frame #4 {
                                n3537 = Multiply(x="delay s", y=u32 1000) -> (x*y=w1846:u32)
                                n3538 = Wait (ms)(milliseconds to wait=w1846) -> ()  [unwired: 1 out]
                                }
                                }
                                }
                                frame True {
                                n3539 = flat-sequence {
                                tunnel: w1851 -> [w1852]
                                tunnel: w1850 -> [w1860]
                                tunnel: [w1866] -> w1849
                                tunnel: w1849 -> [w1869]
                                frame #0 {
                                n3540 = local read "control hz array"() -> (w1855:dbl[][])
                                n3541 = call "change2d.vi"("reset(default false)"=TRUE, "index (col)"=w1852, "index (row)"=1, "read/write(T/F)"=FALSE, "2D Array"=w1855) -> ("2D Array Result"=w1856:dbl[][])  [unwired: 5 in, 1 out]
                                n3542 = local write "control hz array"(w1856) -> ()
                                }
                                frame #1 {
                                n3543 = Wait (ms)(milliseconds to wait=u32 500) -> ()  [unwired: 1 out]
                                }
                                frame #2 {
                                n3544 = local read "control hz array"() -> (w1863:dbl[][])
                                n3545 = local write "frekans index"(0.0 ("frekans index")) -> ()
                                n3546 = call "change2d.vi"("reset(default false)"=FALSE, "index (col)"=w1860, "index (row)"=2, "read/write(T/F)"=FALSE, "2D Array"=w1863) -> ("2D Array Result"=w1864:dbl[][])  [unwired: 5 in, 1 out]
                                n3547 = local write "control hz array"(w1864) -> ()
                                }
                                frame #3 {
                                n3548 = One Button Dialog(message="SECTIGINIZ FREKANSLAR DENGELENDI\n1- Ana Program sekmesinden hata veren frekans varsa bakabilirsiniz\n2- Excel çıktılarını kaydetmeyi unutmayınız\n**Hata kodu verirse önemsemeyiniz**", button name ("OK")="TAMAM") -> (true=w1866:bool)
                                }
                                frame #4 {
                                n3549 = case shown="False" w1869 {
                                frame False {
                                n3550 = local write "stop listbox"(TRUE ("stop listbox")) -> ()
                                n3551 = local write "Stop"(TRUE ("Stop")) -> ()
                                }
                                frame True {
                                n3552 = local write "stop listbox"(TRUE ("stop listbox")) -> ()
                                n3553 = local write "Stop"(TRUE ("Stop")) -> ()
                                }
                                }
                                }
                                }
                                }
                                }
                              }
                            }
                          }
                        }
                      }
